vi "tcsWEP_logEvent_famTargetWfsList.vi"(8 "error in (no error)":errorcluster, 11 "logevent_famTargetWfsList_Ctl":T1={"sensorIdList[189]"=[0, 0, 0, 0, 0, 0, 0, 0, 0, 0, 0, 0, 0, 0, 0, 0, 0, 0, 0, 0, 0, 0, 0, 0, 0, 0, 0, 0, 0, 0, 0, 0, 0, 0, 0, 0, 0, 0, 0, 0, 0, 0, 0, 0, 0, 0, 0, 0, 0, 0, 0, 0, 0, 0, 0, 0, 0, 0, 0, 0, 0, 0, 0, 0, 0, 0, 0, 0, 0, 0, 0, 0, 0, 0, 0, 0, 0, 0, 0, 0, 0, 0, 0, 0, 0, 0, 0, 0, 0, 0, 0, 0, 0, 0, 0, 0, 0, 0, 0, 0, 0, 0, 0, 0, 0, 0, 0, 0, 0, 0, 0, 0, 0, 0, 0, 0, 0, 0, 0, 0, 0, 0, 0, 0, 0, 0, 0, 0, 0, 0, 0, 0, 0, 0, 0, 0, 0, 0, 0, 0, 0, 0, 0, 0, 0, 0, 0, 0, 0, 0, 0, 0, 0, 0, 0, 0, 0, 0, 0, 0, 0, 0, 0, 0, 0, 0, 0, 0, 0, 0, 0, 0, 0, 0, 0, 0, 0, 0, 0, 0, 0, 0, 0, 0, 0, 0, 0, 0, 0], "timestamp"=0.0, "priority"=0}) -> (0 "error out":errorcluster, 2 "function return":i32, 3 "logevent_famTargetWfsList_Ctl out":T1)   [LabVIEW 2016, in "SALLV_tcsWEP.lvlib"]
doc: "int tcsWEP_shm_logEvent_famTargetWfsListLV(tcsWEP_logevent_famTargetWfsListLV *logevent_famTargetWfsList_Ctl );"
uses:
  SALLV_tcsWEP.lvlib
  DataTypes/logevent_famTargetWfsList.ctl
  SALLV_tcsWEP.so
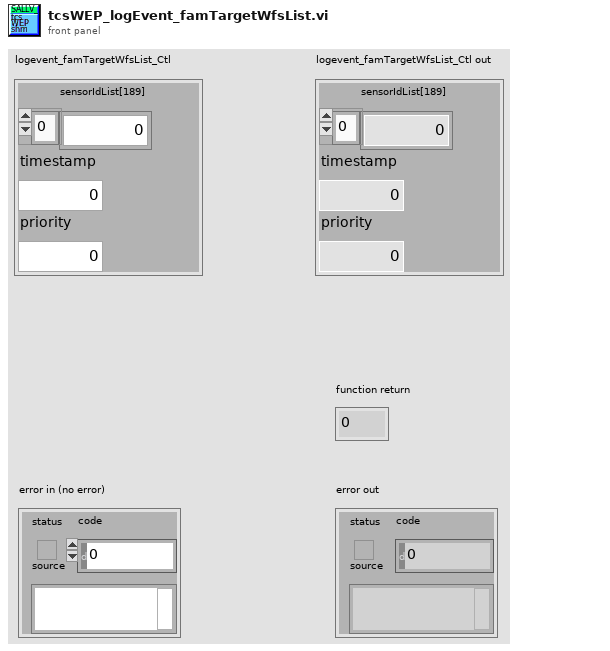
[diagram p1: front panel]
types:
  T1 = typedef "SALLV_tcsWEP.lvlib/logevent_famTargetWfsList.ctl" = cluster{"sensorIdList[189]":i16[], "timestamp":dbl, "priority":i32}
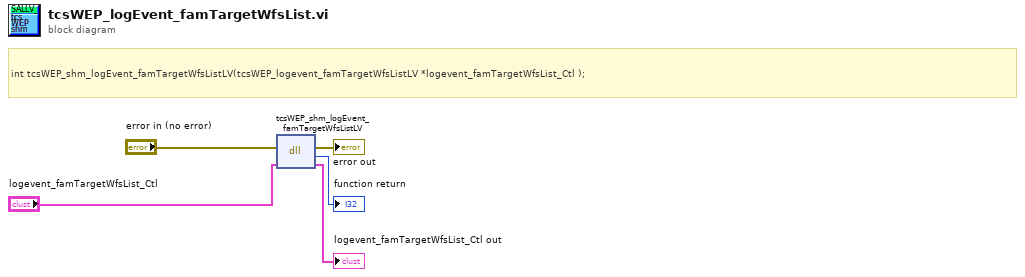
[diagram p0: block diagram]
diagram:
  # "int tcsWEP_shm_logEvent_famTargetWfsListLV(tcsWEP_logevent_famTargetWfsListLV *logevent_famTargetWfsList_Ctl );"
  n1 = dll-call lib="home/ttsai/Documents/salAPI/SALLV_tcsWEP.*" fn="tcsWEP_shm_logEvent_famTargetWfsListLV"(error in="error in (no error)", "logevent_famTargetWfsList_Ctl"="logevent_famTargetWfsList_Ctl") -> (error out=→"error out":errorcluster, →"function return":i32, "logevent_famTargetWfsList_Ctl"=→"logevent_famTargetWfsList_Ctl out":T1)  [unwired: 2 in, 1 out]
